vi "Start Data Viewer.vi"(10 "Results":refnum<vi>, 11 "Application in":refnum<class "Application.lvclass">) -> (0 "error out":errorcluster, 3 "Data Viewer out":refnum<class "Data Viewer.lvclass">)   [LabVIEW 2017, in "Application.lvlib" / "Application.lvclass"]
doc: "Initializes the DataViewer object inside the application."
uses:
  Application.lvclass
  <vilib>/TSS/ACRObat Test Framework/Classes/Data/Data Viewer/Class/Data Viewer.lvclass
  C:/Program Files (x86)/National Instruments/LabVIEW 2017/vi.lib/TSS/ACRObat Test Framework/Classes/Base Objects/Base Class/Base Class/Base Class.lvclass
  <vilib>/TSS/ACRObat Test Framework/Classes/Base Objects/Base Class/Base Class/Base Class.lvclass
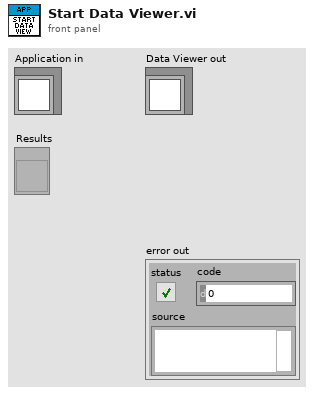
[diagram p1: front panel]
types:
  T1 = typedef "Application.lvlib/App Settings.lvclass/Class Settings -- Cluster.ctl" = cluster{"DataLogging Enabled":bool, "AutoStart":bool, "AutoClear":bool, "Cycle Timeout":u32, "Wait Before Clear":u32, "Machine ID":string, "Test Type":string, "Product Name":string, "Meta Tags":string[], "Meta Values":string[], "Viewer Settings":cluster{"DataViewer Headers":string[], "Pass Fail Settings":T2}}
  T2 = typedef "Data Viewer.lvlib/Data Viewer Settings.lvclass/Pass Fail Criteria -- Cluster.ctl" = cluster{"Header":string, "Criteria":string}
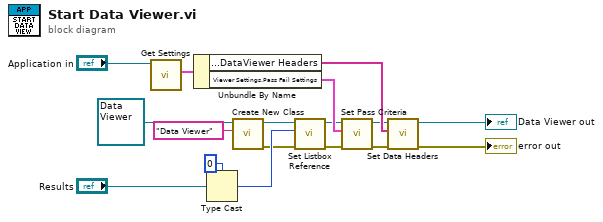
[diagram p0: block diagram]
diagram:
  n1 = call "Get Settings.vi"("Acrobat Template in"="Application in") -> ("Settings"=w15:T1)  [unwired: 8 in, 2 out]
  n2 = Unbundle By Name(w15) -> ("Viewer Settings.DataViewer Headers"=w17:string[], "Viewer Settings.Pass Fail Settings"=w16:T2)
  n3 = Type Cast(type=0 ("Listbox Reference"), x="Results") -> (*(type *) &x=w12:i32)
  n4 = call <vilib>:"Create New Class.vi"("Name"="Data Viewer", "Base Class in"=refnum<class "Data Viewer.lvclass"> refnum ("Acrobat Template in")) -> ("error out"=w11:errorcluster, "Base Class out"=w2:refnum<class "Data Viewer.lvclass">)  [unwired: 8 in]
  n5 = call <vilib>:"Set Listbox Reference.vi"("error in (no error)"=w11, "Listbox Reference"=w12, "Acrobat Template in"=w2) -> ("error out"=w8:errorcluster, "Acrobat Template out"=w7:refnum<class "Data Viewer.lvclass">)  [unwired: 7 in]
  n6 = call <vilib>:"Set Pass Criteria.vi"("error in (no error)"=w8, "Pass Fail Settings"=w16, "Acrobat Template in"=w7) -> ("error out"=w9:errorcluster, "Acrobat Template out"=w6:refnum<class "Data Viewer.lvclass">)  [unwired: 7 in]
  n7 = call <vilib>:"Set Data Headers.vi"("error in (no error)"=w9, "Headers"=w17, "Acrobat Template in"=w6) -> ("error out"=→"error out":errorcluster, "Acrobat Template out"=→"Data Viewer out":refnum<class "Data Viewer.lvclass">)  [unwired: 7 in]
